vi "Read TestLogFactory.vi"(11 "Model in":refnum<class "Model.lvclass">) -> (2 "ITestLogFactory.lvclass":refnum<class "ITestLogFactory.lvclass">, 3 "Model out":refnum<class "Model.lvclass">)   [LabVIEW 2015, in "Model.lvclass"]
uses:
  Model.lvclass
  TestLogFactory/ITestLogFactory/ITestLogFactory.lvclass
  Model.lvclass/Model.ctl
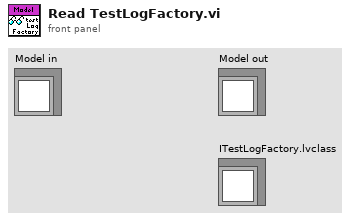
[diagram p1: front panel]
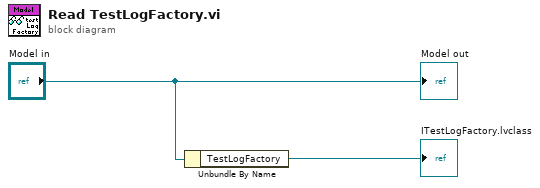
[diagram p0: block diagram]
diagram:
  n1 = Unbundle By Name("Model in") -> ("TestLogFactory"=→"ITestLogFactory.lvclass":refnum<class "ITestLogFactory.lvclass">)
  "Model out" <- "Model in"
